vi "Set PSU Voltage.vi"(4 "error in":errorcluster, 6 "Voltage":dbl format="%0.2f") -> (0 "error out":errorcluster)   [LabVIEW 2015]
uses:
  <vilib>/DAQmx/write.llb/DAQmx Write (Analog DBL 1Chan 1Samp).vi
  <vilib>/DAQmx/miscellaneous.llb/DAQmx Fill In Error Info.vi
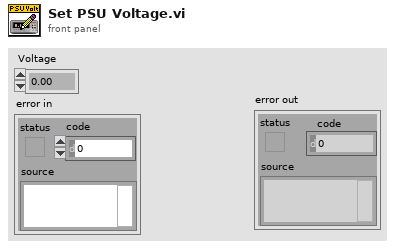
[diagram p1: front panel]
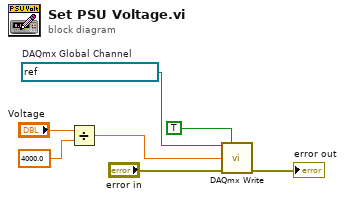
[diagram p0: block diagram]
diagram:
  w7 = refnum<k21> "AO0 PSU Voltage Set"  # DAQmx Global Channel
  n1 = Divide(x="Voltage", y=4000.0) -> (x/y=w1:dbl)
  n2 = call-poly <vilib>:"DAQmx Write.vi"("task/channels in"=w7, "auto start"=TRUE, "data"=w1, "error in"="error in") -> ("error out"=→"error out":errorcluster)  [unwired: 9 in, 2 out]
